vi "Set Intensity Graph Y Scale Min and Max.vi"(8 "error in (no error)":errorcluster, 9 "End [1]":dbl=1.0, 10 "Start [0]":dbl, 11 "graph_utilities in":refnum<class "graph_utilities.lvclass">) -> (0 "error out":errorcluster, 3 "graph_utilities out":refnum<class "graph_utilities.lvclass">)   [LabVIEW 2019, in "graph_utilities.lvclass"]
doc: "Set the Y Offset and Multiple of the Intensity Graph by wiring an array to Y Scale"
uses:
  graph_utilities.lvclass
  <vilib>/Utility/miscctls.llb/LVOffsetAndMultiplierTypeDef.ctl
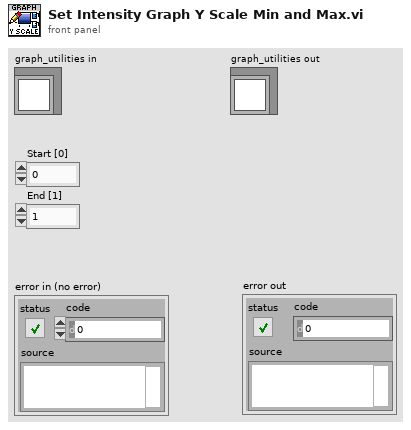
[diagram p1: front panel]
types:
  T1 = typedef "LVOffsetAndMultiplierTypeDef.ctl" = cluster{"Offset":dbl, "Multiplier":dbl}
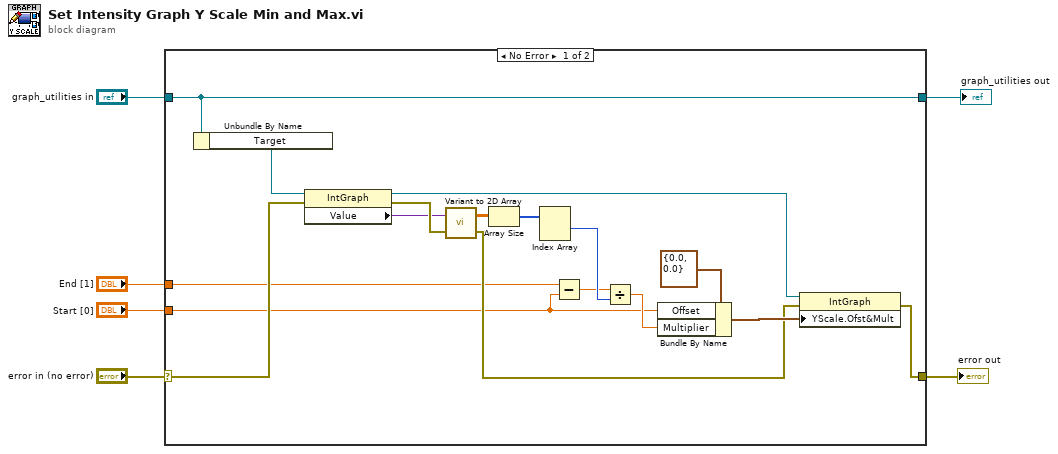
[diagram p0: block diagram]
diagram:
  n1 = case shown="No Error" "error in (no error)" {
    selector: "error in (no error)" -> [w13 w25]
    tunnel: [w7 w25] -> w6
    tunnel: "graph_utilities in" -> [w23 w24]
    tunnel: [w23 w24] -> w3
    tunnel: "End [1]" -> [w9 _]
    tunnel: "Start [0]" -> [w8 _]
    frame No Error {
      n2 = Unbundle By Name(w23) -> ("Target"=w14:refnum<vi>)
      n3 = property on="Property Node" class="IntGraph"(reference=w14, error in=w13) -> (reference out=w10:refnum<vi>, error out=w20:errorcluster, "Value"=w19:variant)
      n4 = call "Variant to 2D Array.vi"("error in (no error)"=w20, "Value"=w19) -> ("error out"=w11:errorcluster, "Array"=w21:dbl[][])
      n5 = Array Size(array=w21) -> (size(s)=w22:i32[])
      n6 = Index Array(array=w22) -> (element #1=w18:i32)  [unwired: 2 in, 1 out]
      n7 = Subtract(x=w9, y=w8) -> (x-y=w15:dbl)
      n8 = Divide(x=w15, y=w18) -> (x/y=w17:dbl)
      n9 = Bundle By Name(cluster=T1 {"Offset"=0.0, "Multiplier"=0.0} ("X Scale.Offset and Multiplier"), "Offset"=w8, "Multiplier"=w17) -> (w12:T1)
      n10 = property on="Property Node" class="IntGraph"(reference=w10, error in=w11, "YScale.Ofst&Mult"=w12) -> (error out=w7:errorcluster)  [unwired: 1 out]
    }
    frame Error {
    }
  }
  "error out" <- w6
  "graph_utilities out" <- w3
